vi "Change Process Params.vi"(8 "error in (no error)":errorcluster, 10 "New Params":T1={"Mode"=enum."ROI", "Manual LUT"={"Minimum"=0.0, "Maximum"=0.0}, "BCG Values"={"Brightness"=128.0, "Contrast"=45.0, "Gamma"=1.0}, "Log?"=FALSE, "Auto?"=FALSE, "ROI"={"Global Rectangle"=[], "Contours"=[]}, "Image X"=0, "Image Y"=0, "HROI Pos"=0}, 11 "CameraPreview in":refnum<class "CameraPreview.lvclass">) -> (0 "error out":errorcluster, 3 "CameraPreview out":refnum<class "CameraPreview.lvclass">)   [LabVIEW 2023, in "CameraPreview.lvlib" / "CameraPreview.lvclass"]
uses:
  CameraPreview.lvclass
  typedefs/ImageProcessingParametersInPreview.ctl
  CameraPreview.lvclass/CameraPreview.ctl
  <vilib>/vision/NI_Vision_Development_Module.lvlib
  Camera_Controller/Camera_Controller.lvlib
  typedefs/typedefs.lvlib
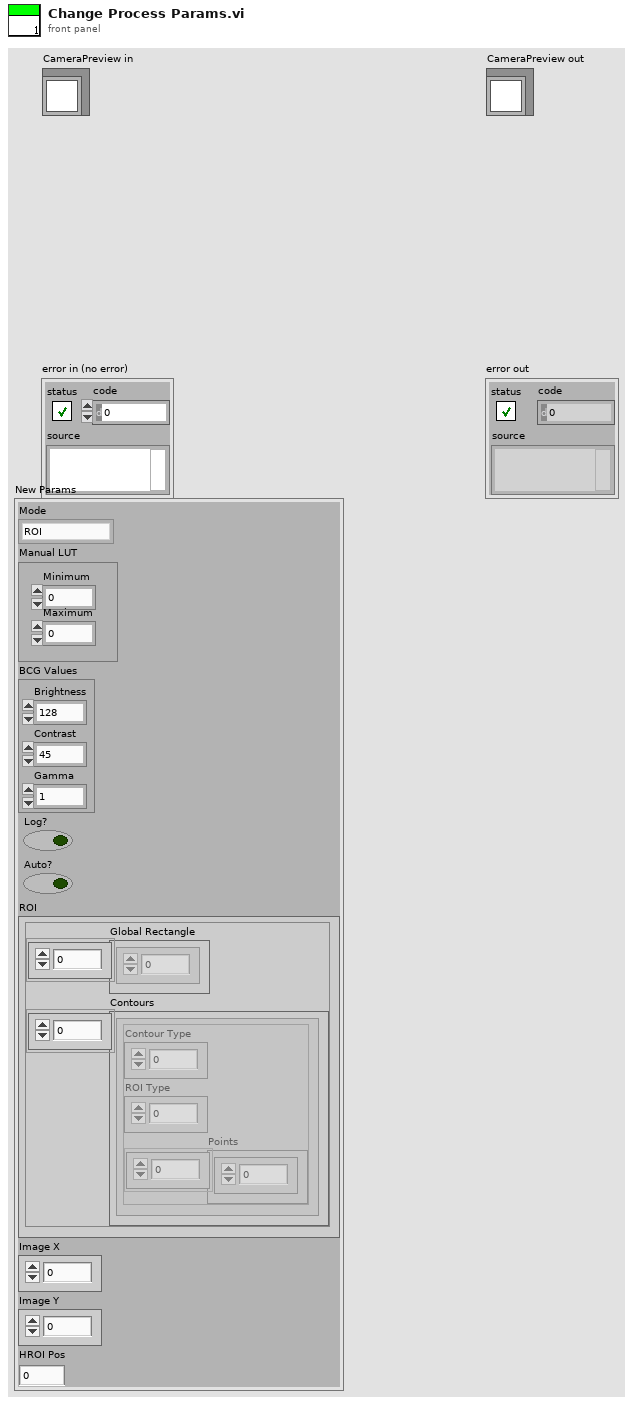
[diagram p1: front panel]
types:
  T1 = typedef "typedefs.lvlib/ImageProcessingParametersInPreview.ctl" = cluster{"Mode":enum16{"ROI", "Image"}, "Manual LUT":cluster{"Minimum":dbl, "Maximum":dbl}, "BCG Values":cluster{"Brightness":sgl, "Contrast":sgl, "Gamma":sgl}, "Log?":bool, "Auto?":bool, "ROI":cluster{"Global Rectangle":i32[], "Contours":cluster{"Contour Type":u32, "ROI Type":u32, "Points":i32[]}[]}, "Image X":i32, "Image Y":i32, "HROI Pos":u16}
  T2 = enum32{"Linear", "Log", "Exp", "Square", "Square root", "Power X", "Power 1/X"}
  T3 = typedef "IMAQ Image.ctl" = refnum<image>
  T4 = cluster{"Brightness":sgl, "Contrast":sgl, "Gamma":sgl}
  T5 = cluster{"Lower value":sgl, "Upper value":sgl, "Replace Value":sgl, "Keep/Replace Value (Replace)":bool}[]
  T6 = cluster{"Global Rectangle":i32[], "Contours":cluster{"Contour Type":u32, "ROI Type":u32, "Points":i32[]}[]}
  T7 = cluster{"Min":sgl, "Max":sgl, "Mean":sgl, "Std Dev":sgl, "Count":i32, "Size (um)":i32}
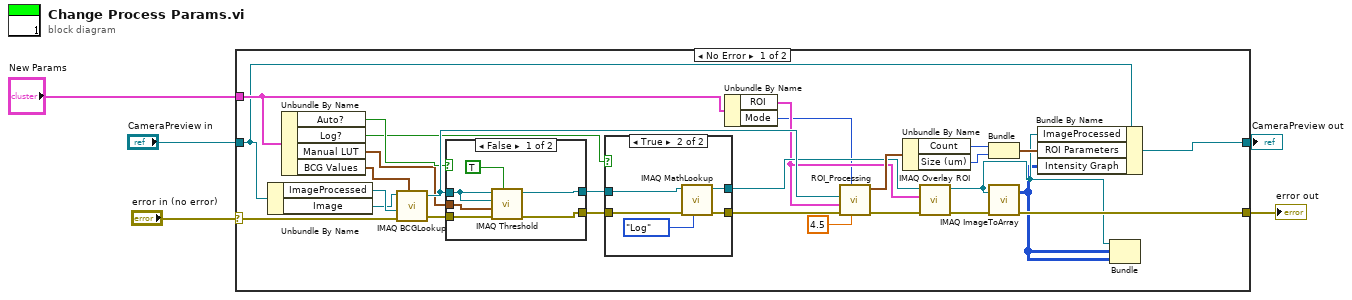
[diagram p0: block diagram]
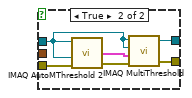
[diagram p3: hidden frame]
diagram:
  n1 = case shown="No Error" "error in (no error)" {
    selector: "error in (no error)" -> [w15 w54]
    tunnel: [w14 w54] -> w4
    tunnel: [w9 w53] -> w2
    tunnel: "CameraPreview in" -> [w11 w53]
    tunnel: "New Params" -> [w13 _]
    frame No Error {
      n2 = Unbundle By Name(w11) -> ("ImageProcessed"=w12:T3, "Image"=w10:T3)
      n3 = Unbundle By Name(w13) -> ("Auto?"=w25:bool, "Log?"=w22:bool, "Manual LUT"=w24:cluster{"Minimum":dbl, "Maximum":dbl}, "BCG Values"=w23:T4)
      n4 = call "IMAQ BCGLookup"("Image Src"=w10, "BCG Values"=w23, "Image Dst"=w12, "error in (no error)"=w15) -> ("Image Dst Out"=w32:T3, "error out"=w31:errorcluster)  [unwired: 3 in]
      n5 = case shown="False" w25 {
        tunnel: w32 -> [w42 w50]
        tunnel: [w44 w49] -> w29
        tunnel: w31 -> [w46 w52]
        tunnel: [w45 w47] -> w30
        tunnel: w24 -> [w43 _]
        frame False {
          n6 = call "IMAQ Threshold"("Keep/Replace Value (Replace)"=TRUE, "error in (no error)"=w46, "Range"=w43, "Image Dst"=w42, "Image Src"=w42) -> ("error out"=w45:errorcluster, "Image Dst Out"=w44:T3)  [unwired: 5 in]
        }
        frame True {
          n7 = call "IMAQ AutoMThreshold 2"("error in (no error)"=w52, "Image Mask"=w50, "Image"=w50) -> ("error out"=w48:errorcluster, "Threshold Data out"=w51:T5)  [unwired: 1 in, 1 out]
          n8 = call "IMAQ MultiThreshold"("error in (no error)"=w48, "Threshold Data"=w51, "Image Dst"=w50, "Image Src"=w50) -> ("error out"=w47:errorcluster, "Image Dst Out"=w49:T3)  [unwired: 1 in]
        }
      }
      n9 = case shown="True" w22 {
        tunnel: w29 -> [w34 w39]
        tunnel: w30 -> [w35 w38]
        tunnel: [w35 w37] -> w21
        tunnel: [w34 w36] -> w20
        frame False {
        }
        frame True {
          n10 = call "IMAQ MathLookup"("Operator"=T2."Log", "error in (no error)"=w38, "Image Src"=w39) -> ("error out"=w37:errorcluster, "Image Dst Out"=w36:T3)  [unwired: 7 in]
        }
      }
      n11 = Unbundle By Name(w13) -> ("ROI"=w17:T6, "Mode"=w16:enum16{"ROI", "Image"})
      n12 = call "ROI_Processing.vi"("Pixel Size(um)"=4.5, "Histogram Mode"=w16, "error in (no error)"=w21, "ROI"=w17, "Image Dst Out"=w32) -> ("error out"=w19:errorcluster, "ROI Pixel Statistics"=w26:T7)  [unwired: 4 in, 1 out]
      n13 = Unbundle By Name(w26) -> ("Count"=w27:i32, "Size (um)"=w28:i32)
      n14 = call "IMAQ Overlay ROI"("error in (no error)"=w19, "ROI Descriptor"=w17, "Image"=w20) -> ("error out"=w18:errorcluster, "Image Out"=w7:T3)  [unwired: 7 in]
      n15 = Bundle("Count"=w27, "Size (um)"=w28) -> (w8:cluster{"Count":i32, "Size (um)":i32})  [unwired: 1 in]
      n16 = call "IMAQ ImageToArray"("error in (no error)"=w18, "Image"=w7) -> ("error out"=w14:errorcluster, "Image Pixels (U8)"=w6:u8[][])  [unwired: 2 in, 3 out]
      n17 = Bundle By Name(cluster=w11, "ImageProcessed"=w7, "ROI Parameters"=w8, "Intensity Graph"=w6) -> (w9:refnum<class "CameraPreview.lvclass">)
      n18 = Bundle("Image Out"=w7, "Image Pixels (U8)"=w6, "Image Pixels (U8)"=w6) -> ()  [unwired: 1 in, 1 out]
    }
    frame Error {
    }
  }
  "error out" <- w4
  "CameraPreview out" <- w2
